vi "Illini Hyperloop GUI v4.0.vi"() -> ()   [LabVIEW 2015]
uses:
  <vilib>/robotics/Controls/Attitude Indicator/Attitude Indicator.xctl
  CommunicationStatus.ctl
  StageEnum.ctl
  ArxPaxGauge4.ctl
  MicrosecondsGauge1.ctl
  <vilib>/Analysis/Matrix/Datatypes/RealMatrix.ctl
  <vilib>/Analysis/NI_AALBase.lvlib
  <vilib>/Analysis/Matrix/NI_Matrix.lvlib
panel:
  out "X acc":dbl
  out "Acceleration Chart":dbl(graph)
  out "A * B 2":T1
  in  "Reset Sensor":bool
  out "Current State:":string
  in  "Transition to:":string(combo)="Safe Mode"
  in  "Transition":bool
  in  "VR3":dbl
  in  "VR2":dbl
  in  "VR1":dbl
  in  "VL3":dbl
  in  "VL2":dbl
  in  "VL1":dbl
  out "RPM Right Front":T2 scale=0.0..6000.0
  out "RPM Right Mid":T2 scale=0.0..6000.0
  out "LEV Micro":T3 scale=800.0..2000.0
  out "RPM Right Back":T2 scale=0.0..6000.0
  out "RPM Left Front":T2 scale=0.0..6000.0
  out "RPM Left Mid":T2 scale=0.0..6000.0
  out "LEV  Delay timer":dbl
  out "STA  Delay timer":dbl
  out "Battery Pack 2 V 2":dbl(slide) caption="Capacity %" scale=0.0..100.0
  out "Battery Pack 1 V 2":dbl(slide) caption="Capacity %" scale=0.0..100.0
  out "Battery Pack 2 V":dbl(slide) caption="Pack 2 (V)" scale=0.0..500.0
  out "Battery Pack 1 V":dbl(slide) caption="Pack 1 (V)" scale=0.0..500.0
  out "Levitation Chart":cluster{"element":dbl, "element":dbl}(graph)
  out "Braking Force Chart 1":dbl(slide) caption="Reservoir 1" scale=0.0..6000.0
  out "Levitation height front":dbl(slide) caption="Front" scale=0.0..20.0
  out "Levitation height back":dbl(slide) caption="Back" scale=0.0..20.0
  out "Attitude Indicator":cluster{"Roll":dbl, "Pitch":dbl}(xcontrol)
  out "Yaw":dbl(knob) scale=-15.0..15.0
  out "RPM Left Back":T2 scale=0.0..6000.0
  out "Cabin Pressure":dbl format="%#.3g"
  out "Ambient Pressure (psi)":dbl(graph)
  out "Pod State:":T4
  out "Communication Status:":T5=enum."Disconnected"
  out "Low Battery":dbl format="%#.2g"
  out "High Battery:":dbl format="%#.2g"
  out "Battery 3":dbl(slide) scale=0.0..100.0
  out "Battery 2":dbl(slide) scale=0.0..100.0
  out "Battery 1":dbl(slide) scale=0.0..100.0
  out "Z vel":dbl
  out "Y vel":dbl
  out "X vel":dbl
  out "Z position":dbl
  out "Y pos":dbl
  out "X pos":dbl
  out "Velocity Chart":dbl(graph)
  in  "EMERGENCY BRAKE":bool
  in  "Functional Test Tab Control":T6(tab)
  out "Client Closed":string="The client VI closed the connection."
  out "Most Recent Data":string
  in  "Connect to":string="192.168.137.10"
  in  "timeout ms":i32=1000
  in  "port":u16=8888
  in  "ms per loop":u32
  in  "bytes per write":i32=1000
  out "Base File Name":string
  in  "Stop Program":bool
  out "Producer Error Messages":errorcluster
  out "Consumer Error Messages":errorcluster
  in  "LEV OFF 2":bool
  in  "LEV ON 2":bool
  in  "LEV OFF":bool
  in  "STA Delay":dbl=100.0
  in  "LEV Delay":dbl=100.0
  in  "STA Start Stop":bool
  in  "LEV Start Stop":bool
  in  "STA jump Interval":dbl=5.0
  in  "STA Target":dbl=1000.0
  in  "LEV jump interval":dbl=5.0
  in  "LEV Target":dbl=1000.0
  in  "LEV ON":bool
  in  "SET STA Manual":bool
  in  "Set LEV Manual":bool
  in  "LEV SLIDE":dbl(slide) scale=0.0..2000.0
  in  "STA Slide":dbl(slide) scale=0.0..2000.0
  in  "STA Margin":dbl=50.0
  in  "LEV Margin":dbl=50.0
  in  "Stop":bool
  in  "Backward":bool
  in  "Forward":bool
  out "Status ERROR":string caption="Data:"
  out "Status Messages":string caption="Data:"
  out "Status STATE&CONTROL":string caption="Data:"
  in  "Prepare for Launch":bool caption="Boolean"
  out "Checkmark":u16(ring)
  out "Position Chart":dbl(graph)
  out "Temperature other (C)":T7(graph)
  out "Temperature ESCs (C)":T8(graph)
  # "Illini Hyperloop"
  # "Brakes (PSI)"
  # "X Position (m)"
  # "Levitation (m)"
  # "Levitation (mm)"
  # "Attitude"
  # "X Acceleration (g)"
  # "X Velocity (m/s)"
  # "Levitation Battery Packs"
  # "Motor Control"
  # "Brake Control"
  # "MESSAGE"
  # "ERROR"
  # "STATE & CONTROL"
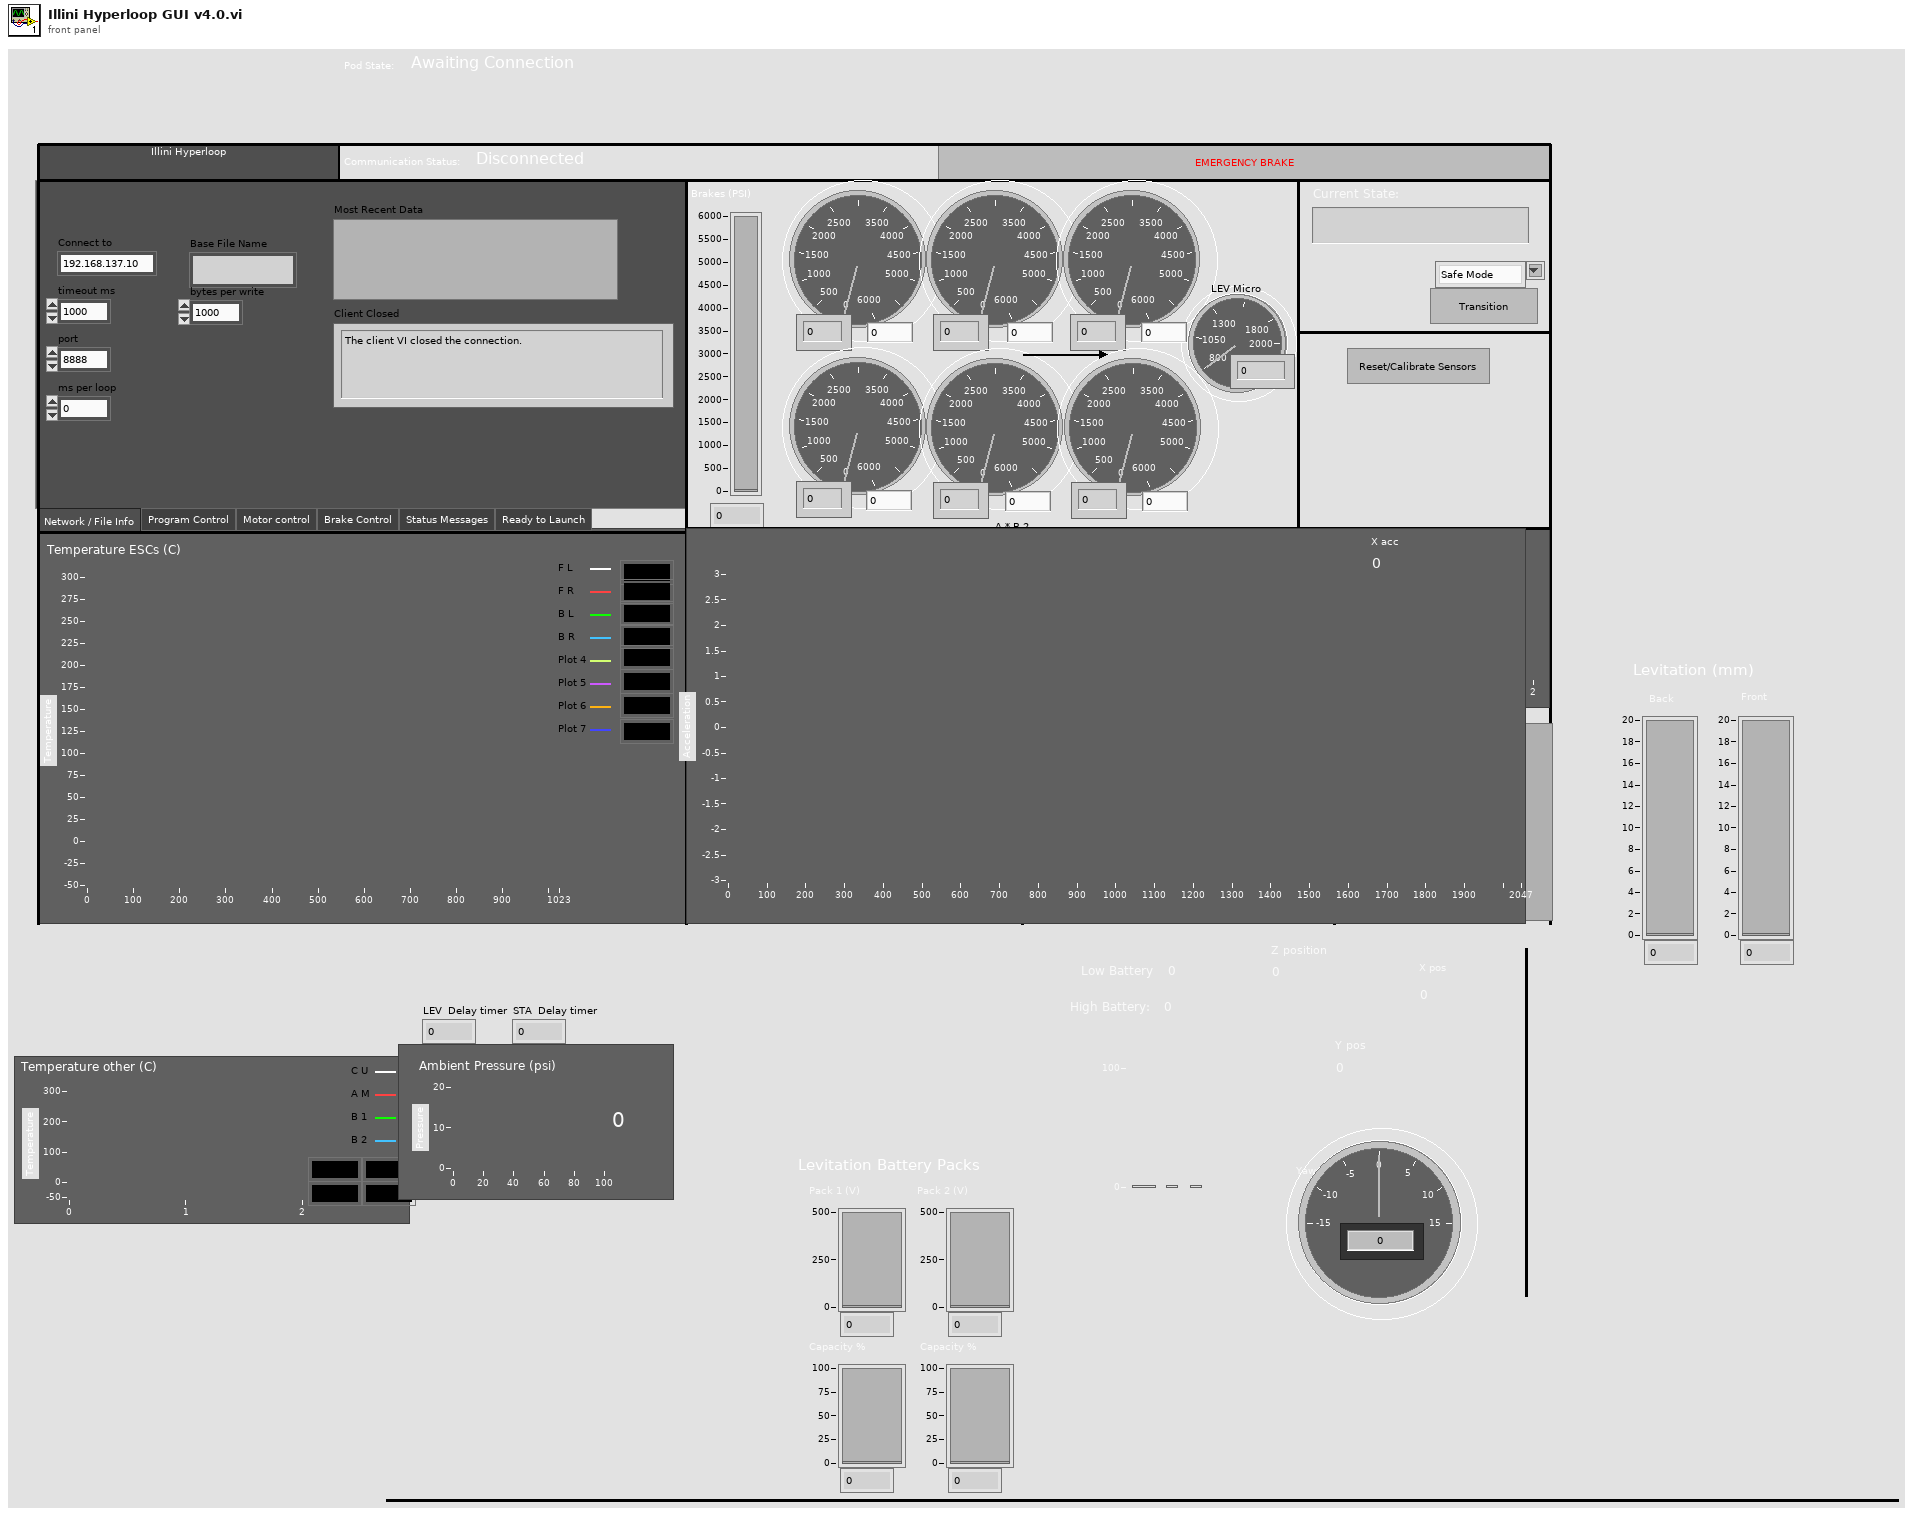
[diagram p1: front panel]
types:
  T1 = typedef "NI_Matrix.lvlib/RealMatrix.ctl" = dbl[][]
  T2 = typedef "ArxPaxGauge4.ctl" = u32
  T3 = typedef "MicrosecondsGauge1.ctl" = dbl
  T4 = typedef "StageEnum.ctl" = enum16{"Awaiting Connection", "TEST Comms", "TEST Lev", "TEST Inside Comms", "TEST Internal Power", "Ready to Launch", "Acceleration", "Coast", "Brake"}
  T5 = typedef "CommunicationStatus.ctl" = enum16{"Connected", "Disconnected"}
  T6 = enum32{"Network / File Info", "Program Control", "Motor control", "Brake Control", "Status Messages", "Ready to Launch"}
  T7 = cluster{"element":dbl, "element":dbl, "element":dbl, "element":dbl}
  T8 = cluster{"element":dbl, "element":dbl, "element":dbl, "element":dbl, "element":dbl, "element":dbl, "element":dbl, "element":dbl}
  T9 = cluster{"element":dbl, "element":dbl, "element":dbl, "element":dbl, "element":dbl, "element":dbl, "element":dbl, "element":dbl}[]
  T10 = cluster{"element":dbl, "element":dbl, "element":dbl, "element":dbl}[]
  T11 = enum16{"Standard", "Buffered", "CRLF", "Immediate"}
  T12 = cluster{i32, "data out":string, "data out":string}
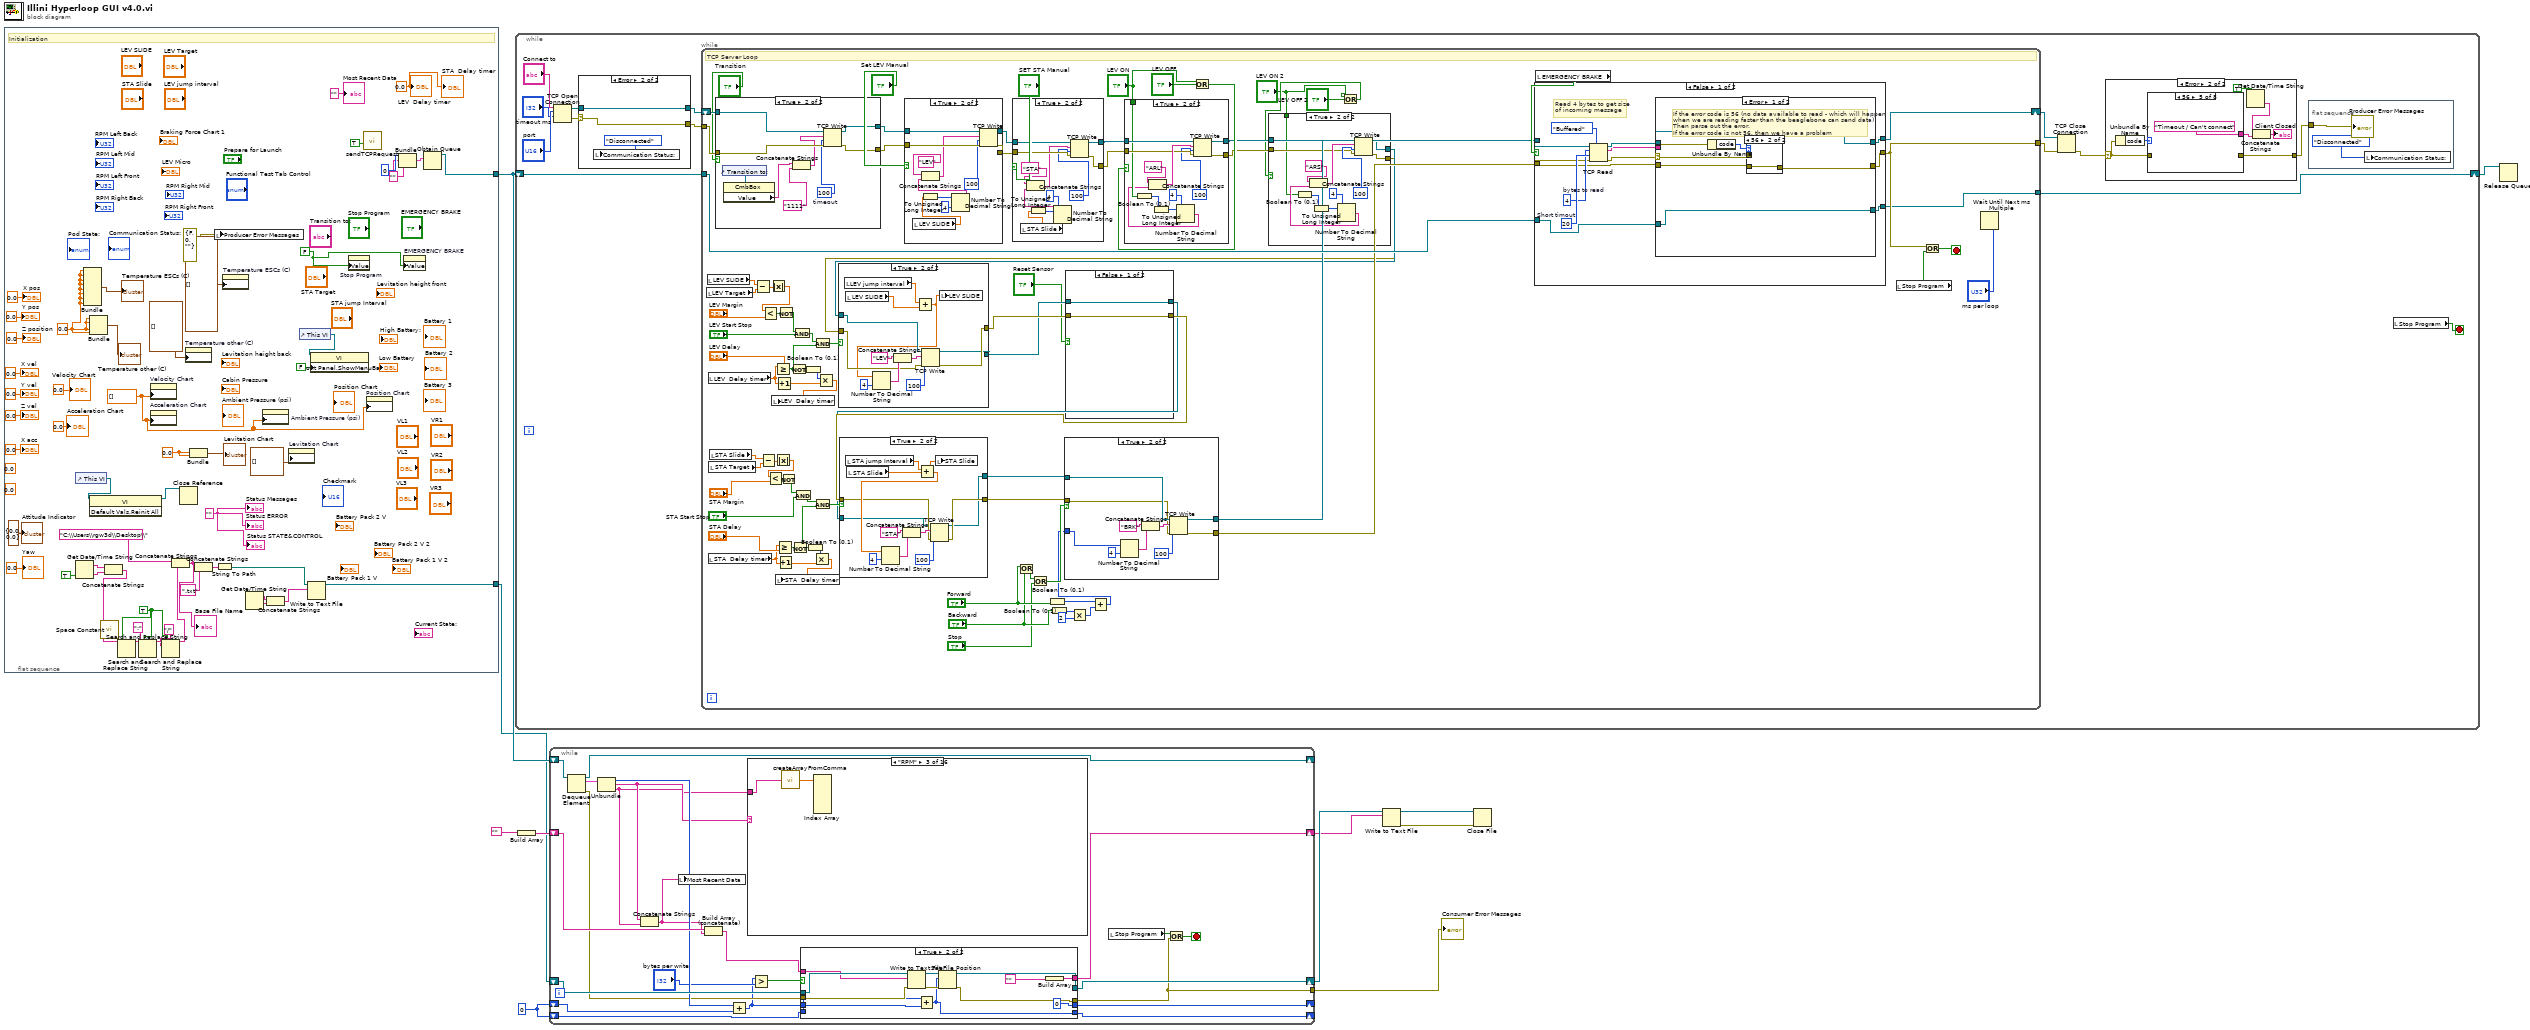
[diagram p0: block diagram]
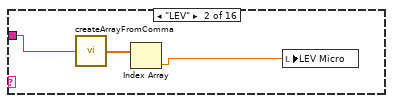
[diagram p4: hidden frame]
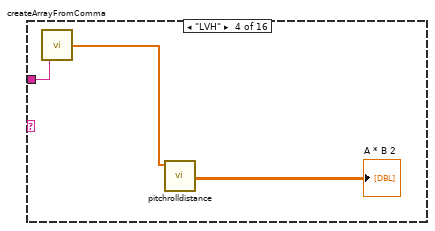
[diagram p5: hidden frame]
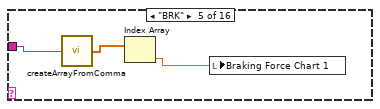
[diagram p6: hidden frame]
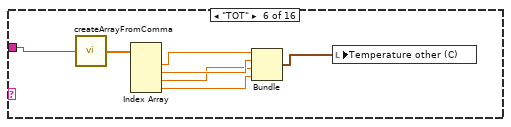
[diagram p7: hidden frame]
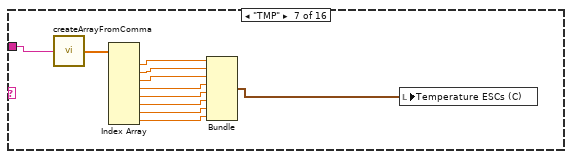
[diagram p8: hidden frame]
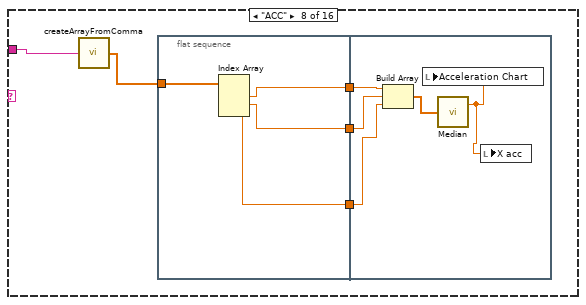
[diagram p9: hidden frame]
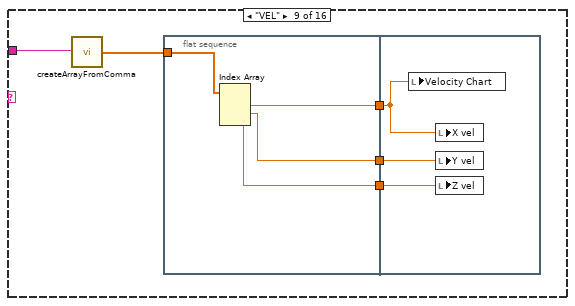
[diagram p10: hidden frame]
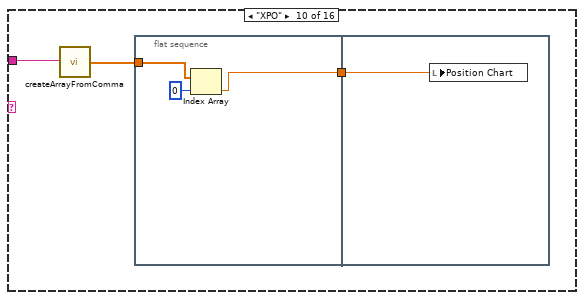
[diagram p11: hidden frame]
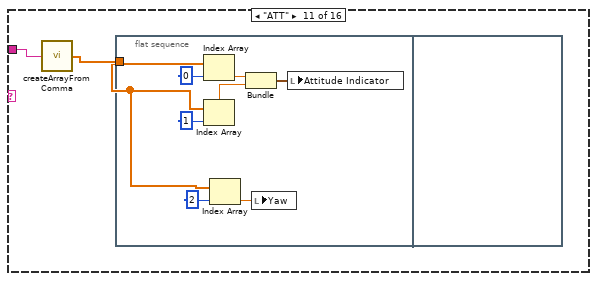
[diagram p12: hidden frame]
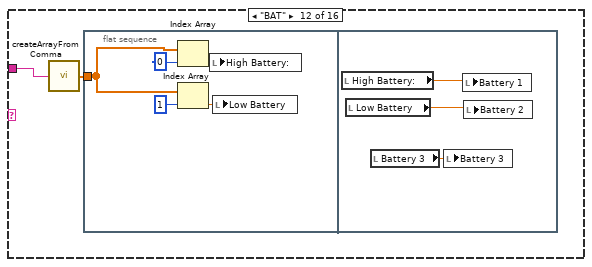
[diagram p13: hidden frame]
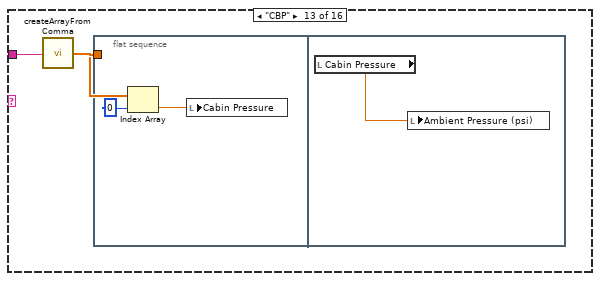
[diagram p14: hidden frame]
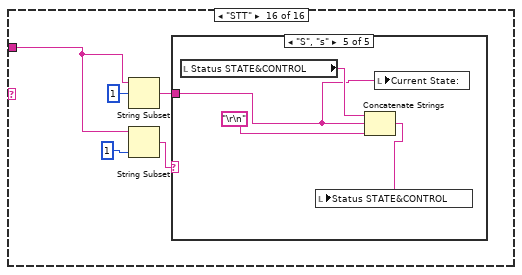
[diagram p17: hidden frame]
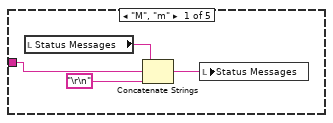
[diagram p18: hidden frame]
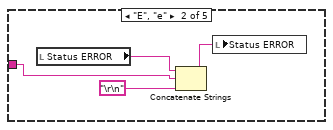
[diagram p19: hidden frame]
diagram:
  w1 = 0
  n1 = flat-sequence {
    tunnel: [w65] -> w11
    tunnel: [w40] -> w6
    frame #0 {
      w20 = 0.0 ("LEV  Delay timer")
      w23 = 0.0 ("element")
      w24 = TRUE ("want seconds? (F)")
      w37 = ""
      w44 = dbl[] [] ("History Data")
      w19 = 0.0 ("element")
      w52 = FALSE
      w12 = "" ("Functional Test 1 Data")
      (unwired) 0.0 ("Y acceleration")
      (unwired) 0.0 ("Z acceleration")
      # "Initialization"
      n2 = control-ref of="This VI"() -> (w46:refnum<vi>)
      n3 = Get Date/Time String(want seconds? (F)=TRUE) -> (date string=w35:string, time string=w34:string)  [unwired: 2 in]
      n4 = Bundle("element"=w19, "element"=w19, "element"=w19, "element"=w19, "element"=w19, "element"=w19, "element"=w19, "element"=w19) -> (→"Temperature ESCs (C)":T8)  [unwired: 1 in]
      n5 = Bundle("element"=w19, "element"=w19, "element"=w19, "element"=w19) -> (→"Temperature other (C)":T7)  [unwired: 1 in]
      n6 = invoke class="VI" method="Default Vals.Reinit All"(reference=w46) -> (reference out=w45:refnum<vi>)  [unwired: 2 in, 2 out]
      n7 = call <vilib>:"Space Constant.vi"() -> ("String"=w36:string)
      n8 = Concatenate Strings(w35, w34) -> (w33:string)
      n9 = Search and Replace String(replace all?=w24, input string=w33, search string=w36) -> (result string=w31:string)  [unwired: 5 in, 3 out]
      n10 = Search and Replace String(replace all?=w24, input string=w31, search string=":" ("Functional Test 1 Data")) -> (result string=w27:string)  [unwired: 5 in, 3 out]
      n11 = property on="Velocity Chart" class="WFChart (strict)"("History Data"=w44) -> ()  [unwired: 2 in, 2 out]
      n12 = property on="Acceleration Chart" class="WFChart (strict)"("History Data"=w44) -> ()  [unwired: 2 in, 2 out]
      n13 = Search and Replace String(replace all?=w24, input string=w27, search string="/" ("Functional Test 1 Data")) -> (result string=w26:string)  [unwired: 5 in, 3 out]
      n14 = Concatenate Strings("C:\\Users\\rgw3d\\Desktop\\" ("Functional Test 1 Data"), w26) -> (w14:string)
      "Base File Name" <- w14
      n15 = Close Reference(reference=w45) -> ()  [unwired: 1 in, 1 out]
      n16 = property on="Temperature other (C)" class="WFChart (strict)"("History Data"=T10 []) -> ()  [unwired: 2 in, 2 out]
      n17 = Bundle("element"=w23, "element"=w23) -> (→"Levitation Chart":cluster{"element":dbl, "element":dbl})  [unwired: 1 in]
      n18 = Concatenate Strings(w14, ".txt" ("Functional Test 1 Data")) -> (w15:string)
      n19 = local write "Producer Error Messages"(errorcluster {"status"=FALSE, "code"=0, "source"=""} ("error constant")) -> ()
      n20 = String To Path(string=w15) -> (path=w28:path)
      n21 = property on="Temperature ESCs (C)" class="WFChart (strict)"("History Data"=T9 []) -> ()  [unwired: 2 in, 2 out]
      n22 = Get Date/Time String() -> (date string=w43:string, time string=w42:string)  [unwired: 3 in]
      n23 = property on="Ambient Pressure (psi)" class="WFChart (strict)"("History Data"=w44) -> ()  [unwired: 2 in, 2 out]
      n24 = Concatenate Strings(w43, w42) -> (w41:string)
      n25 = property on="Levitation Chart" class="WFChart (strict)"("History Data"=cluster{"element":dbl, "element":dbl}[] []) -> ()  [unwired: 2 in, 2 out]
      n26 = control-ref of="This VI"() -> (w51:refnum<vi>)
      n27 = Write to Text File(file (use dialog)=w28, text=w41) -> (refnum out=w40:refnum<file>)  [unwired: 2 in, 2 out]
      n28 = property class="VI"(reference=w51, "Front Panel.ShowMenuBar"=FALSE ("Front Panel Window:Show Menu Bar")) -> ()  [unwired: 1 in, 2 out]
      n29 = property on="Stop Program" class="Bool (strict)"("Value"=w52) -> ()  [unwired: 2 in, 2 out]
      n30 = call "sendTCPRequest.vi"("Force Reset"=TRUE) -> ()  [unwired: 9 in, 2 out]
      n31 = property on="Position Chart" class="WFChart (strict)"("History Data"=w44) -> ()  [unwired: 2 in, 2 out]
      n32 = Bundle(0, w37, w37) -> (w39:cluster{i32, string, string})  [unwired: 1 in]
      n33 = property on="EMERGENCY BRAKE" class="Bool (strict)"("Value"=w52) -> ()  [unwired: 2 in, 2 out]
      n34 = Obtain Queue(element data type=w39) -> (queue out=w65:refnum<queue>)  [unwired: 4 in, 2 out]
      "X pos" <- 0.0 ("X position")
      "Y pos" <- 0.0 ("Y position")
      "Z position" <- 0.0 ("Z position")
      "X vel" <- 0.0 ("X velocity")
      "Y vel" <- 0.0 ("Y velocity")
      "Z vel" <- 0.0 ("Z velocity")
      "X acc" <- 0.0 ("X acceleration")
      "Velocity Chart" <- 0.0 ("Velocity (m/s)")
      "Attitude Indicator" <- cluster{"Roll":dbl, "Pitch":dbl} {"Roll"=0.0, "Pitch"=0.0} ("Attitude Indicator")
      "Acceleration Chart" <- 0.0 ("Acceleration Chart")
      "Yaw" <- 0.0 ("Yaw")
      "Status Messages" <- w12
      "Most Recent Data" <- "" ("Data out")
      "LEV  Delay timer" <- w20
      "STA  Delay timer" <- w20
      "Status ERROR" <- w12
      "Status STATE&CONTROL" <- w12
    }
  }
  n35 = while {
    shift-right: [w72] -> w10
    shift-left: w11 -> [w73]
    stop <- w69 stop-if-true
    n36 = TCP Open Connection(address="Connect to", remote port or service name="port", timeout ms (60000)="timeout ms") -> (connection ID=w74:refnum<k5>, error out=w75:errorcluster)  [unwired: 2 in]
    n37 = case shown="Error" w75 {
      selector: w75 -> [_ w85]
      tunnel: w74 -> [w83 w86]
      tunnel: [w83 w86] -> w67
      tunnel: [_ w85] -> w66
      frame No Error {
        # "No error.. \nwe connected!"
        n38 = local write "Communication Status:"(CommunicationStatus."Connected" ("Communication Status")) -> ()
      }
      frame Error {
        n39 = local write "Communication Status:"(CommunicationStatus."Disconnected" ("Communication Status")) -> ()
      }
    }
    n40 = while {
      tunnel: w66 -> [w178]
      tunnel: [w183] -> w71
      tunnel: w73 -> [w173]
      tunnel: [w182] -> w72
      shift-right: [w181] -> w68
      shift-left: w67 -> [w179]
      stop <- w172 stop-if-true
      # "TCP Server Loop"
      n41 = local read "LEV Target"() -> (w167:dbl)
      n42 = local read "LEV SLIDE"() -> (w168:dbl)
      n43 = local read "LEV  Delay timer"() -> (w155:dbl)
      n44 = local read "STA  Delay timer"() -> (w154:dbl)
      n45 = local read "STA Target"() -> (w161:dbl)
      n46 = local read "STA Slide"() -> (w162:dbl)
      n47 = case shown="True" "Transition" {
        tunnel: w179 -> [w294 w303]
        tunnel: w178 -> [w293 w301]
        tunnel: [w293 w300] -> w176
        tunnel: [w294 w302] -> w174
        frame False {
        }
        frame True {
          w299 = 100  # timeout
          n48 = control-ref of="Transition to:"() -> (w298:refnum<vi>)
          n49 = property class="CmbBox"(reference=w298) -> ("Value"=w297:string)  [unwired: 1 in, 2 out]
          n50 = Concatenate Strings(w297, "1111") -> (w295:string)
          n51 = TCP Write(connection ID=w303, data in=w295, error in (no error)=w301, 9:w299) -> (connection ID out=w302:refnum<k5>, error out=w300:errorcluster)  [unwired: 1 out]
        }
      }
      n52 = Subtract(x=w168, y=w167) -> (x-y=w166:dbl)
      n53 = Subtract(x=w162, y=w161) -> (x-y=w164:dbl)
      n54 = Absolute Value(x=w166) -> (abs(x)=w165:dbl)
      n55 = Less?(x=w165, y="LEV Margin") -> (x < y?=w146:bool)
      n56 = Greater Or Equal?(x=w155, y="LEV Delay") -> (x >= y?=w143:bool)
      n57 = Absolute Value(x=w164) -> (abs(x)=w163:dbl)
      n58 = Less?(x=w163, y="STA Margin") -> (x < y?=w137:bool)
      n59 = Increment(x=w155) -> (x+1=w152:dbl)
      n60 = Greater Or Equal?(x=w154, y="STA Delay") -> (x >= y?=w135:bool)
      n61 = Increment(x=w154) -> (x+1=w140:dbl)
      n62 = Not(x=w146) -> (.not. x?=w144:bool)
      n63 = Not(x=w137) -> (.not. x?=w138:bool)
      n64 = Not(x=w143) -> (.not. x?=w153:bool)
      n65 = Not(x=w135) -> (.not. x?=w148:bool)
      n66 = And(x=w144, y="LEV Start Stop") -> (x .and. y?=w142:bool)
      n67 = And(x=w138, y="STA Start Stop") -> (x .and. y?=w158:bool)
      n68 = Boolean To (0,1)(Boolean=w153) -> (0, 1=w150:i16)
      n69 = Boolean To (0,1)(Boolean=w148) -> (0, 1=w147:i16)
      n70 = Multiply(x=w147, y=w140) -> (x*y=w149:dbl)
      n71 = local write "STA  Delay timer"(w149) -> ()
      n72 = And(x=w142, y=w143) -> (x .and. y?=w156:bool)
      n73 = And(x=w158, y=w135) -> (x .and. y?=w157:bool)
      n74 = Multiply(x=w150, y=w152) -> (x*y=w151:dbl)
      n75 = local write "LEV  Delay timer"(w151) -> ()
      n76 = case shown="True" "Set LEV Manual" {
        tunnel: w176 -> [w280 w292]
        tunnel: [w280 w291] -> w170
        tunnel: w174 -> [w281 w290]
        tunnel: [w281 w289] -> w171
        frame False {
        }
        frame True {
          n77 = local read "LEV SLIDE"() -> (w283:dbl)
          n78 = To Unsigned Long Integer(number=w283) -> (unsigned 32bit integer=w282:u32)
          n79 = Number To Decimal String(number=w282, width (-)=i16 4) -> (decimal integer string=w286:string)
          n80 = Concatenate Strings("LEV", w286) -> (w285:string)
          n81 = TCP Write(connection ID=w290, data in=w285, error in (no error)=w292, 9:100 ("timeout ms (25000)")) -> (connection ID out=w289:refnum<k5>, error out=w291:errorcluster)  [unwired: 1 out]
        }
      }
      n82 = case shown="True" "SET STA Manual" {
        tunnel: w171 -> [w268 w279]
        tunnel: [w268 w278] -> w134
        tunnel: w170 -> [w267 w277]
        tunnel: [w267 w276] -> w133
        frame False {
        }
        frame True {
          n83 = local read "STA Slide"() -> (w269:dbl)
          n84 = To Unsigned Long Integer(number=w269) -> (unsigned 32bit integer=w270:u32)
          n85 = Number To Decimal String(number=w270, width (-)=i16 4) -> (decimal integer string=w273:string)
          n86 = Concatenate Strings("STA", w273) -> (w272:string)
          n87 = TCP Write(connection ID=w279, data in=w272, error in (no error)=w277, 9:100 ("timeout ms (25000)")) -> (connection ID out=w278:refnum<k5>, error out=w276:errorcluster)  [unwired: 1 out]
        }
      }
      n88 = Or(x="Forward", y="Backward") -> (x .or. y?=w127:bool)
      n89 = Or(x=w127, y="Stop") -> (x .or. y?=w126:bool)
      n90 = Boolean To (0,1)(Boolean="Forward") -> (0, 1=w120:i16)
      n91 = Boolean To (0,1)(Boolean="Backward") -> (0, 1=w122:i16)
      n92 = Multiply(x=w122, y=i16 2) -> (x*y=w119:i16)
      n93 = Add(x=w120, y=w119) -> (x+y=w118:i16)
      n94 = Or(x="LEV ON", y="LEV OFF") -> (x .or. y?=w131:bool)
      n95 = case shown="True" w131 {
        tunnel: w134 -> [w225 w235]
        tunnel: w133 -> [w226 w234]
        tunnel: [w226 w233] -> w113
        tunnel: [w225 w232] -> w114
        tunnel: "LEV ON" -> [_ w229]
        frame False {
        }
        frame True {
          n96 = Boolean To (0,1)(Boolean=w229) -> (0, 1=w230:i16)
          n97 = To Unsigned Long Integer(number=w230) -> (unsigned 32bit integer=w236:u32)
          n98 = Number To Decimal String(number=w236, width (-)=i16 4) -> (decimal integer string=w227:string)
          n99 = Concatenate Strings("ARL", w227) -> (w238:string)
          n100 = TCP Write(connection ID=w235, data in=w238, error in (no error)=w234, 9:100 ("timeout ms (25000)")) -> (connection ID out=w232:refnum<k5>, error out=w233:errorcluster)  [unwired: 1 out]
        }
      }
      n101 = Or(x="LEV ON 2", y="LEV OFF 2") -> (x .or. y?=w112:bool)
      n102 = case shown="True" w112 {
        tunnel: w114 -> [w200 w206]
        tunnel: w113 -> [w199 w205]
        tunnel: [w200 w204] -> w111
        tunnel: [w199 w203] -> w110
        tunnel: "LEV ON 2" -> [_ w201]
        frame False {
        }
        frame True {
          n103 = Boolean To (0,1)(Boolean=w201) -> (0, 1=w208:i16)
          n104 = To Unsigned Long Integer(number=w208) -> (unsigned 32bit integer=w210:u32)
          n105 = Number To Decimal String(number=w210, width (-)=i16 4) -> (decimal integer string=w202:string)
          n106 = Concatenate Strings("ARS", w202) -> (w212:string)
          n107 = TCP Write(connection ID=w206, data in=w212, error in (no error)=w205, 9:100 ("timeout ms (25000)")) -> (connection ID out=w204:refnum<k5>, error out=w203:errorcluster)  [unwired: 1 out]
        }
      }
      n108 = case shown="True" w156 {
        tunnel: w111 -> [w254 w260]
        tunnel: [w254 w256] -> w107
        tunnel: w110 -> [w253 w259]
        tunnel: [w253 w258] -> w108
        frame False {
        }
        frame True {
          n109 = local read "LEV jump interval"() -> (w266:dbl)
          n110 = local read "LEV SLIDE"() -> (w265:dbl)
          n111 = Add(x=w266, y=w265) -> (x+y=w257:dbl)
          n112 = Number To Decimal String(number=w257, width (-)=i16 4) -> (decimal integer string=w262:string)
          n113 = Concatenate Strings("LEV", w262) -> (w264:string)
          n114 = TCP Write(connection ID=w260, data in=w264, error in (no error)=w259, 9:100 ("timeout ms (25000)")) -> (connection ID out=w256:refnum<k5>, error out=w258:errorcluster)  [unwired: 1 out]
          n115 = local write "LEV SLIDE"(w257) -> ()
        }
      }
      n116 = case shown="False" "Reset Sensor" {
        tunnel: w108 -> [w186 w193]
        tunnel: w107 -> [w187 w192]
        tunnel: [w186 w189] -> w106
        tunnel: [w187 w188] -> w105
        frame False {
        }
        frame True {
          n117 = To Unsigned Long Integer(number=0) -> (unsigned 32bit integer=w198:u32)
          n118 = Number To Decimal String(number=w198, width (-)=i16 4) -> (decimal integer string=w195:string)
          n119 = Concatenate Strings("RST", w195) -> (w196:string)
          n120 = TCP Write(connection ID=w192, data in=w196, error in (no error)=w193, 9:100 ("timeout ms (25000)")) -> (connection ID out=w188:refnum<k5>, error out=w189:errorcluster)  [unwired: 1 out]
        }
      }
      n121 = case shown="True" w157 {
        tunnel: w106 -> [w240 w244]
        tunnel: [w240 w243] -> w129
        tunnel: w105 -> [w239 w242]
        tunnel: [w239 w241] -> w128
        frame False {
        }
        frame True {
          n122 = local read "STA jump Interval"() -> (w252:dbl)
          n123 = local read "STA Slide"() -> (w251:dbl)
          n124 = Add(x=w252, y=w251) -> (x+y=w245:dbl)
          n125 = Number To Decimal String(number=w245, width (-)=i16 4) -> (decimal integer string=w248:string)
          n126 = Concatenate Strings("STA", w248) -> (w250:string)
          n127 = TCP Write(connection ID=w242, data in=w250, error in (no error)=w244, 9:100 ("timeout ms (25000)")) -> (connection ID out=w241:refnum<k5>, error out=w243:errorcluster)  [unwired: 1 out]
          n128 = local write "STA Slide"(w245) -> ()
        }
      }
      n129 = case shown="True" w126 {
        tunnel: w129 -> [w214 w217]
        tunnel: w128 -> [w213 w218]
        tunnel: w118 -> [_ w219]
        tunnel: [w214 w216] -> w117
        tunnel: [w213 w215] -> w116
        frame False {
        }
        frame True {
          n130 = Number To Decimal String(number=w219, width (-)=i16 4) -> (decimal integer string=w222:string)
          n131 = Concatenate Strings("BRK", w222) -> (w224:string)
          n132 = TCP Write(connection ID=w218, data in=w224, error in (no error)=w217, 9:100 ("timeout ms (25000)")) -> (connection ID out=w215:refnum<k5>, error out=w216:errorcluster)  [unwired: 1 out]
        }
      }
      n133 = local read "EMERGENCY BRAKE"() -> (w185:bool)
      n134 = case shown="False" w185 {
        tunnel: w117 -> [w312 w337]
        tunnel: w116 -> [w313 w336]
        tunnel: [w309 w335] -> w181
        tunnel: [w305 w334] -> w183
        tunnel: w173 -> [w307 w333]
        tunnel: [w306 w333] -> w182
        frame False {
          w314 = 4  # bytes to read
          w315 = 20  # Short timout
          # "Read 4 bytes to get size\nof incoming message"
          n135 = TCP Read(connection ID=w313, bytes to read=w314, error in (no error)=w312, 7:T11."Buffered" ("mode (standard)"), 9:w315) -> (connection ID out=w310:refnum<k5>, data out=w308:string, error out=w311:errorcluster)
          n136 = case shown="Error" w311 {
            selector: w311 -> [w319 _]
            tunnel: w312 -> [w320 w330]
            tunnel: [w318 w325] -> w305
            tunnel: w310 -> [w317 w331]
            tunnel: [w317 w329] -> w309
            tunnel: w308 -> [_ w332]
            tunnel: w307 -> [w316 w327]
            tunnel: [w316 w324] -> w306
            frame Error {
              # "If the error code is 56 (no data available to read - which will happen when we are reading faster than the beaglebone can send data) Then parse out the error. \nIf the error code is not 56, then we have a problem"
              n137 = Unbundle By Name(w319) -> ("code"=w321:i32)
              n138 = case shown="56" w321 {
                tunnel: w319 -> [w322 _]
                tunnel: [w322 w323] -> w318
                tunnel: w320 -> [_ w323]
                frame Default {
                }
                frame 56 {
                }
              }
            }
            frame No Error {
              n139 = call "readTCPDataIn v1.vi"("TCP Network Connection in"=w331, "Size of data"=w332, "error in (no error)"=w330) -> ("TCP Network Connection out"=w329:refnum<k5>, "Size+Operation+Data"=w328:T12, "error out"=w326:errorcluster)  [unwired: 8 in, 2 out]
              n140 = Enqueue Element(queue=w327, element=w328, error in (no error)=w326) -> (queue out=w324:refnum<queue>, error out=w325:errorcluster)  [unwired: 1 in, 1 out]
            }
          }
        }
        frame True {
          n141 = TCP Write(connection ID=w336, data in="OFF0000", error in (no error)=w337) -> (connection ID out=w335:refnum<k5>, error out=w334:errorcluster)  [unwired: 1 in, 1 out]
        }
      }
      n142 = local read "Stop Program"() -> (w184:bool)
      n143 = Or(x=w183, y=w184) -> (x .or. y?=w172:bool)
      n144 = Wait Until Next ms Multiple(millisecond multiple="ms per loop") -> ()  [unwired: 1 out]
    }
    n145 = TCP Close Connection(connection ID=w68, error in (no error)=w71) -> (error out=w79:errorcluster)  [unwired: 2 out]
    n146 = case shown="Error" w79 {
      selector: w79 -> [w87 w93]
      tunnel: [w87 w92] -> w78
      frame No Error {
      }
      frame Error {
        n147 = Unbundle By Name(w93) -> ("code"=w94:i32)
        n148 = case shown="56" w94 {
          tunnel: w93 -> [_ _ w98 _ _ _ _ _]
          tunnel: [_ _ w98 _ _ _ _ _] -> w92
          tunnel: ["The network is down, \nunreachable, or has been reset." "The specified network \naddress is currently in use." "Error" "The system caused the network \nconnection to be aborted." "Timeout / Can't connect" "Error 63. LabVIEW: The network connection \nwas refused by the server." "\tThe network connection\n is not yet established." "The network connection\n was closed by the peer."] -> w89
          frame 59 {
          }
          frame 60 {
          }
          frame Default {
          }
          frame 62 {
          }
          frame 56 {
          }
          frame 63 {
          }
          frame 64 {
          }
          frame 66 {
          }
        }
        n149 = Get Date/Time String(want seconds? (F)=TRUE) -> (time string=w90:string)  [unwired: 2 in, 1 out]
        n150 = Concatenate Strings(w90, w89) -> (→"Client Closed":string)
      }
    }
    n151 = flat-sequence {
      tunnel: w78 -> [w81]
      frame #0 {
        n152 = local write "Communication Status:"(CommunicationStatus."Disconnected" ("Communication Status")) -> ()
        "Producer Error Messages" <- w81
      }
    }
    n153 = local read "Stop Program"() -> (w69:bool)
  }
  n154 = Build Array("") -> (w7:string[])
  n155 = while {
    shift-right: [w361] -> _
    shift-left: w11 -> [w360]
    tunnel: [w349] -> w9
    shift-right: [w341] -> w2
    shift-left: w7 -> [w357]
    shift-right: [w355] -> w5
    shift-left: w6 -> [w356]
    shift-right: [w348] -> _
    shift-left: w1 -> [w352]
    shift-right: [w339] -> _
    shift-left: w1 -> [w340]
    stop <- w358 stop-if-true
    n156 = Dequeue Element(queue=w360) -> (queue out=w361:refnum<queue>, element=w354:cluster{i32, string, string}, error out=w351:errorcluster)  [unwired: 2 in, 1 out]
    n157 = Unbundle(w354) -> (w353:i32, w347:string, w346:string)
    n158 = Concatenate Strings(w347, w346) -> (w344:string)
    n159 = local write "Most Recent Data"(w344) -> ()
    n160 = Build Array (concatenate)(w357, w344) -> (w343:string[])
    n161 = Add(x=w353, y=w352) -> (x+y=w342:i32)
    n162 = case shown="\"RPM\"" w347 {
      tunnel: w346 -> [_ w381 w383 w387 w390 w391 w408 w413 w427 w437 w443 w452 w462 _ _ w471]
      frame Default {
      }
      frame "LEV" {
        n163 = call "createArrayFromComma.vi"("String"=w381) -> ("Array"=w382:dbl[])
        n164 = Index Array(array=w382) -> (element=w380:dbl)  [unwired: 1 in]
        n165 = local write "LEV Micro"(w380) -> ()
      }
      frame "RPM" {
        n166 = call "createArrayFromComma.vi"("String"=w383) -> ("Array"=w384:dbl[])
        n167 = Index Array(array=w384) -> ()  [unwired: 6 in, 6 out]
      }
      frame "LVH" {
        n168 = call "createArrayFromComma.vi"("String"=w387) -> ("Array"=w386:dbl[])
        n169 = call "pitchrolldistance.vi"("input"=w386) -> ("A * B 2"=→"A * B 2":T1)  [unwired: 10 in]
      }
      frame "BRK" {
        n170 = call "createArrayFromComma.vi"("String"=w390) -> ("Array"=w389:dbl[])
        n171 = Index Array(array=w389) -> (element=w388:dbl)  [unwired: 1 in]
        n172 = local write "Braking Force Chart 1"(w388) -> ()
      }
      frame "TOT" {
        n173 = call "createArrayFromComma.vi"("String"=w391) -> ("Array"=w397:dbl[])
        n174 = Index Array(array=w397) -> (element #1=w396:dbl, element #2=w395:dbl, element #3=w394:dbl, element #4=w393:dbl)  [unwired: 4 in]
        n175 = Bundle(w396, w395, w394, w393) -> (w392:cluster{dbl, dbl, dbl, dbl})  [unwired: 1 in]
        n176 = local write "Temperature other (C)"(w392) -> ()
      }
      frame "TMP" {
        n177 = call "createArrayFromComma.vi"("String"=w408) -> ("Array"=w407:dbl[])
        n178 = Index Array(array=w407) -> (element #1=w406:dbl, element #2=w405:dbl, element #3=w403:dbl, element #4=w402:dbl, element #5=w401:dbl, element #6=w400:dbl, element #7=w399:dbl, element #8=w398:dbl)  [unwired: 8 in]
        n179 = Bundle(w406, w405, w403, w402, w401, w400, w399, w398) -> (w404:cluster{dbl, dbl, dbl, dbl, dbl, dbl, dbl, dbl})  [unwired: 1 in]
        n180 = local write "Temperature ESCs (C)"(w404) -> ()
      }
      frame "ACC" {
        n181 = call "createArrayFromComma.vi"("String"=w413) -> ("Array"=w412:dbl[])
        n182 = flat-sequence {
          tunnel: w412 -> [w417]
          tunnel: [w416] -> w411
          tunnel: [w415] -> w410
          tunnel: [w414] -> w409
          tunnel: w411 -> [w422]
          tunnel: w410 -> [w421]
          tunnel: w409 -> [w419]
          frame #0 {
            n183 = Index Array(array=w417) -> (element #1=w416:dbl, element #2=w415:dbl, element #3=w414:dbl)  [unwired: 3 in]
          }
          frame #1 {
            n184 = Build Array(w422, w421, w419) -> (w420:dbl[])
            n185 = call <vilib>:"Median.vi"("X"=w420) -> ("median"=w418:dbl)  [unwired: 1 out]
            n186 = local write "Acceleration Chart"(w418) -> ()
            n187 = local write "X acc"(w418) -> ()
          }
        }
      }
      frame "VEL" {
        n188 = call "createArrayFromComma.vi"("String"=w427) -> ("Array"=w426:dbl[])
        n189 = flat-sequence {
          tunnel: w426 -> [w431]
          tunnel: [w430] -> w425
          tunnel: [w429] -> w424
          tunnel: [w428] -> w423
          tunnel: w425 -> [w434]
          tunnel: w424 -> [w433]
          tunnel: w423 -> [w432]
          frame #0 {
            n190 = Index Array(array=w431) -> (element #1=w430:dbl, element #2=w429:dbl, element #3=w428:dbl)  [unwired: 3 in]
          }
          frame #1 {
            n191 = local write "Velocity Chart"(w434) -> ()
            n192 = local write "X vel"(w434) -> ()
            n193 = local write "Y vel"(w433) -> ()
            n194 = local write "Z vel"(w432) -> ()
          }
        }
      }
      frame "XPO" {
        n195 = call "createArrayFromComma.vi"("String"=w437) -> ("Array"=w436:dbl[])
        n196 = flat-sequence {
          tunnel: w436 -> [w439]
          tunnel: [w438] -> w435
          tunnel: w435 -> [w441]
          frame #0 {
            n197 = Index Array(array=w439, index=0) -> (element=w438:dbl)
          }
          frame #1 {
            n198 = local write "Position Chart"(w441) -> ()
          }
        }
      }
      frame "ATT" {
        n199 = call "createArrayFromComma.vi"("String"=w443) -> ("Array"=w442:dbl[])
        n200 = flat-sequence {
          tunnel: w442 -> [w444]
          frame #0 {
            n201 = Index Array(array=w444, index=0) -> (element=w448:dbl)
            n202 = Index Array(array=w444, index=1) -> (element=w447:dbl)
            n203 = Index Array(array=w444, index=2) -> (element=w445:dbl)
            n204 = Bundle(w448, w447) -> (w446:cluster{dbl, dbl})  [unwired: 1 in]
            n205 = local write "Yaw"(w445) -> ()
            n206 = local write "Attitude Indicator"(w446) -> ()
          }
          frame #1 {
          }
        }
      }
      frame "BAT" {
        n207 = call "createArrayFromComma.vi"("String"=w452) -> ("Array"=w453:dbl[])
        n208 = flat-sequence {
          tunnel: w453 -> [w454]
          frame #0 {
            n209 = Index Array(array=w454, index=0) -> (element=w456:dbl)
            n210 = Index Array(array=w454, index=1) -> (element=w455:dbl)
            n211 = local write "High Battery:"(w456) -> ()
            n212 = local write "Low Battery"(w455) -> ()
          }
          frame #1 {
            n213 = local read "High Battery:"() -> (w460:dbl)
            n214 = local read "Low Battery"() -> (w461:dbl)
            n215 = local read "Battery 3"() -> (w459:dbl)
            n216 = local write "Battery 3"(w459) -> ()
            n217 = local write "Battery 1"(w460) -> ()
            n218 = local write "Battery 2"(w461) -> ()
          }
        }
      }
      frame "CBP" {
        n219 = call "createArrayFromComma.vi"("String"=w462) -> ("Array"=w463:dbl[])
        n220 = flat-sequence {
          tunnel: w463 -> [w465]
          frame #0 {
            n221 = Index Array(array=w465, index=0) -> (element=w464:dbl)
            n222 = local write "Cabin Pressure"(w464) -> ()
          }
          frame #1 {
            n223 = local read "Cabin Pressure"() -> (w467:dbl)
            n224 = local write "Ambient Pressure (psi)"(w467) -> ()
          }
        }
      }
      frame "FAF", "FAT" {
      }
      frame "FBF", "FBT" {
      }
      frame "STT" {
        n225 = String Subset(string=w471, offset (0)=1) -> (substring=w468:string)  [unwired: 1 in]
        n226 = String Subset(string=w471, length (rest)=1 ("length (rest)")) -> (substring=w469:string)  [unwired: 1 in]
        n227 = case shown="\"S\", \"s\"" w469 {
          tunnel: w468 -> [w474 w477 _ w483 w485]
          frame "M", "m" {
            n228 = local read "Status Messages"() -> (w475:string)
            n229 = Concatenate Strings(w475, w474, "\r\n") -> (w476:string)
            n230 = local write "Status Messages"(w476) -> ()
          }
          frame "E", "e" {
            n231 = local read "Status ERROR"() -> (w478:string)
            n232 = Concatenate Strings(w478, w477, "\r\n") -> (w479:string)
            n233 = local write "Status ERROR"(w479) -> ()
          }
          frame Default {
          }
          frame "C", "c" {
            n234 = local read "Status STATE&CONTROL"() -> (w482:string)
            n235 = Concatenate Strings(w482, w483, "\r\n") -> (w481:string)
            n236 = local write "Status STATE&CONTROL"(w481) -> ()
          }
          frame "S", "s" {
            n237 = local read "Status STATE&CONTROL"() -> (w486:string)
            n238 = Concatenate Strings(w486, w485, "\r\n") -> (w487:string)
            n239 = local write "Status STATE&CONTROL"(w487) -> ()
            n240 = local write "Current State:"(w485) -> ()
          }
        }
      }
    }
    n241 = Greater?(x=w342, y="bytes per write") -> (0:w350:bool)
    n242 = case shown="True" w350 {
      tunnel: w343 -> [w363 w370]
      tunnel: w356 -> [w366 w379]
      tunnel: [w366 w373] -> w355
      tunnel: w342 -> [w365 w368]
      tunnel: [w364 w376] -> w349
      tunnel: w351 -> [w364 w375]
      tunnel: [w365 0] -> w348
      tunnel: [w363 w371] -> w341
      tunnel: w340 -> [w362 w369]
      tunnel: [w362 w367] -> w339
      frame False {
      }
      frame True {
        n243 = Write to Text File(file (use dialog)=w379, text=w370, error in=w375) -> (refnum out=w378:refnum<file>, error out=w377:errorcluster)  [unwired: 1 in, 1 out]
        n244 = Add(x=w369, y=w368) -> (x+y=w367:i32)
        n245 = Set File Position(offset (in bytes) (0)=w367, refnum=w378, error in=w377) -> (refnum out=w373:refnum<file>, error out=w376:errorcluster)  [unwired: 1 in]
        n246 = Build Array("") -> (w371:string[])
      }
    }
    n247 = local read "Stop Program"() -> (w359:bool)
    n248 = Or(x=w359, y=w349) -> (x .or. y?=w358:bool)
  }
  "Consumer Error Messages" <- w9
  n249 = Write to Text File(file (use dialog)=w5, text=w2) -> (refnum out=w3:refnum<file>, error out=w4:errorcluster)  [unwired: 2 in, 1 out]
  n250 = Close File(refnum=w3, error in=w4) -> ()  [unwired: 2 out]
  n251 = Release Queue(queue=w10) -> ()  [unwired: 2 in, 3 out]
